vi "Set stack data.vi"(4 "Region":dbl, 6 "Position":dbl, 8 "error in (no error)":errorcluster, 9 "Common data array":string[](array[string]), 10 "Is module?":bool, 11 "Stack in":refnum<class "Stack.lvclass">) -> (0 "error out":errorcluster, 3 "Stack out":refnum<class "Stack.lvclass">)   [LabVIEW 2021, in "Stack.lvclass"]
uses:
  Stack.lvclass
  Stack.lvclass/Stack.ctl
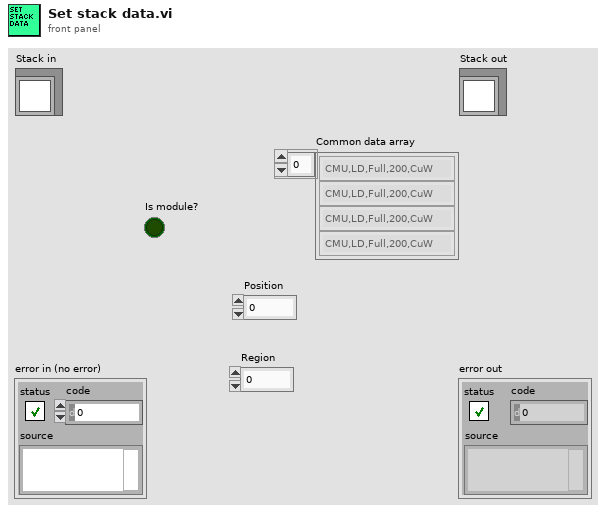
[diagram p1: front panel]
types:
  T1 = cluster{"Common data array[0]":string, "Common data array[1]":string, "Common data array[2]":string, "Common data array[3]":string, "Common data array[4]":string, "Common data array[5]":string, "Common data array[6]":string, "Common data array[7]":string, "Common data array[8]":string}
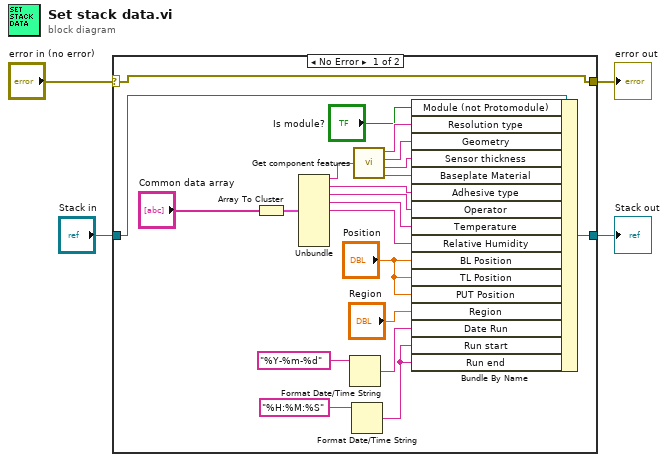
[diagram p0: block diagram]
diagram:
  n1 = case shown="No Error" "error in (no error)" {
    selector: "error in (no error)" -> [w25 w27]
    tunnel: [w25 w27] -> w3
    tunnel: [w24 w26] -> w1
    tunnel: "Stack in" -> [w23 w26]
    frame No Error {
      n2 = Array To Cluster(array="Common data array") -> (cluster=w17:T1)
      n3 = Unbundle(w17) -> ("Common data array[0]"=w16:string, "Common data array[1]"=w15:string, "Common data array[2]"=w14:string, "Common data array[3]"=w12:string, "Common data array[4]"=w13:string)  [unwired: 4 out]
      n4 = Format Date/Time String(time format string (%c)="%Y-%m-%d") -> (date/time string=w6:string)  [unwired: 2 in]
      n5 = Format Date/Time String(time format string (%c)="%H:%M:%S") -> (date/time string=w5:string)  [unwired: 2 in]
      n6 = call "Get component features.vi"("Module Type"=w16) -> ("Resolution"=w21:string, "Geometry"=w22:string, "Sensor thickness"=w20:string, "BP Type"=w19:string)  [unwired: 1 in, 1 out]
      n7 = Bundle By Name(cluster=w23, "Module (not Protomodule)"="Is module?", "Resolution type"=w21, "Geometry"=w22, "Sensor thickness"=w20, "Baseplate Material"=w19, "Adhesive type"=w15, "Operator"=w14, "Temperature"=w12, "Relative Humidity"=w13, "BL Position"="Position", "TL Position"="Position", "PUT Position"="Position", "Region"="Region", "Date Run"=w6, "Run start"=w5, "Run end"=w5) -> (w24:refnum<class "Stack.lvclass">)
    }
    frame Error {
    }
  }
  "error out" <- w3
  "Stack out" <- w1
